vi "log_error.vi"(8 "error in (no error)":errorcluster) -> (0 "error out":errorcluster)   [LabVIEW 2021, in "system.logging.lvclass"]
uses:
  system.logging.lvclass
  system.logging.lvclass/system.logging.ctl
  severity.ctl
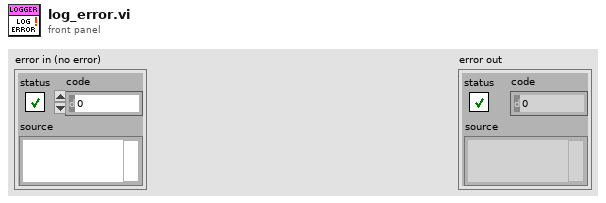
[diagram p1: front panel]
types:
  T1 = typedef "system.logging.lvclass/severity.ctl" = enum8{"trace", "debug", "info", "warning", "error"}
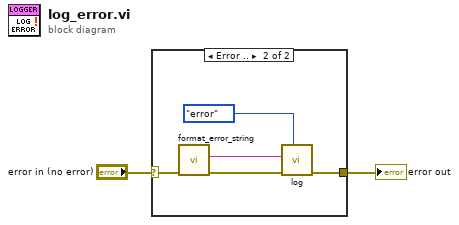
[diagram p0: block diagram]
diagram:
  n1 = case shown="Error .." "error in (no error)" {
    selector: "error in (no error)" -> [w3 w6]
    tunnel: [w3 w8] -> w2
    frame No Error {
    }
    frame Error {
      n2 = call "format_error_string.vi"("error in (no error)"=w6) -> ("error out"=w5:errorcluster, "error_string"=w4:string)  [unwired: 9 in]
      n3 = call "log.vi"("severity"=severity."error", "error in (no error)"=w5, "message"=w4) -> ("error out"=w8:errorcluster)  [unwired: 8 in]
    }
  }
  "error out" <- w2
